vi "plotVesselPosition.vi"(0 "x":dbl, 5 "y":dbl, 7 "angles":dbl[](array[numeric]), 9 "Cluster":cluster{"x":dbl[], "y":dbl[]}, 11 "psi":dbl) -> (8 "XY Graph":cluster{"x":dbl[], "y":dbl[]}[](graph))   [LabVIEW 2014]
uses:
  <vilib>/imath/engines/lvmath2/RunTimeEngine/NodeEndStatement/NIMS_NodeEndStatement_Output.vi
  <instcachedir>/0/NIMS_NodeEndStatement_Output_53EC0D466D134D7ABD903AC30B43404B.lvgen/NIMS_NodeEndStatement_Output_53EC0D466D134D7ABD903AC30B43404B_001.vi
  <vilib>/imath/engines/lvmath2/RunTimeEngine/ErrorHandling/NIMS_Finalize Error.vi
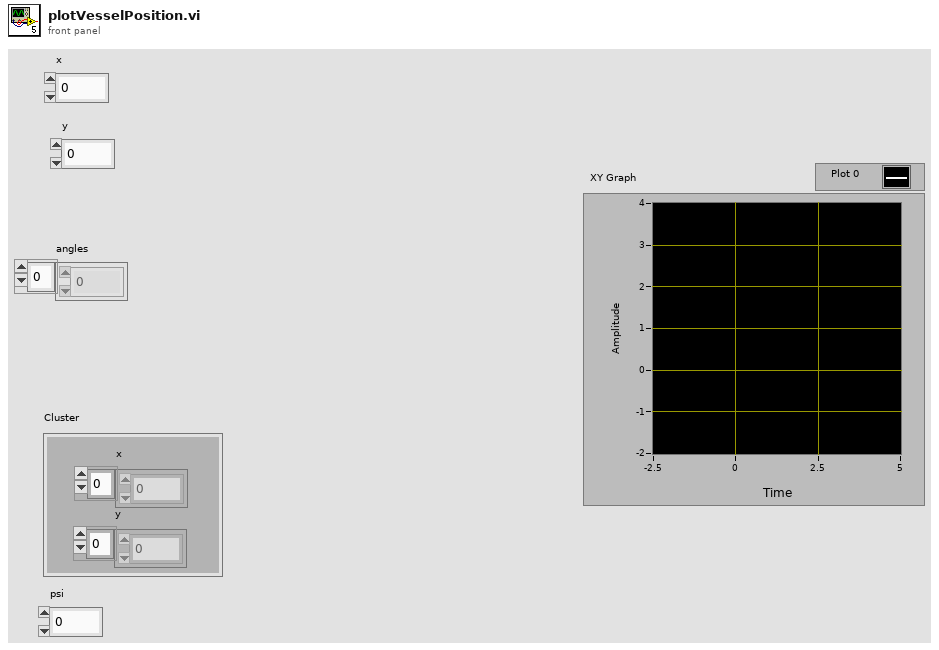
[diagram p1: front panel]
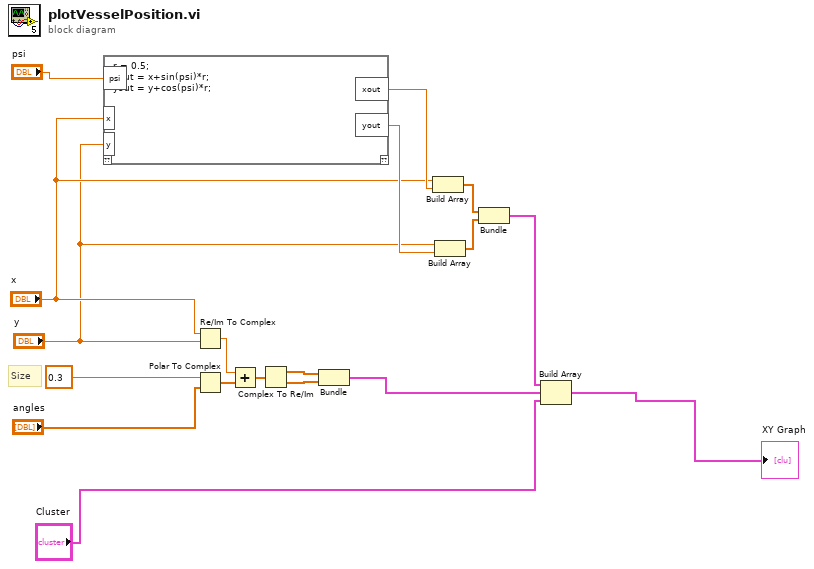
[diagram p0: block diagram]
diagram:
  # "Size"
  n1 = mathscript code="r = 0.5;\nxout = x+sin(psi)*r;\nyout = y+cos(psi)*r;"("x"="x", "y"="y", "psi"="psi") -> ("xout"=w8:dbl, "yout"=w9:dbl)  [unwired: 1 in, 1 out]
  n2 = Re/Im To Complex(1:"y", 2:"x") -> (0:w14:cdb)
  n3 = Polar To Complex(1:"angles", 2:0.3 ("Size")) -> (0:w16:cdb[])
  n4 = Add(x=w14, y=w16) -> (x+y=w15:cdb[])
  n5 = Complex To Re/Im(x + iy=w15) -> (x=w17:dbl[], y=w18:dbl[])
  n6 = Bundle(w17, w18) -> (w11:cluster{dbl[], dbl[]})  [unwired: 1 in]
  n7 = Build Array("x", w8) -> (w2:dbl[])
  n8 = Build Array("y", w9) -> (w1:dbl[])
  n9 = Bundle(w2, w1) -> (w5:cluster{dbl[], dbl[]})  [unwired: 1 in]
  n10 = Build Array(w5, w11, "Cluster") -> (→"XY Graph":cluster{"x":dbl[], "y":dbl[]}[])
